vi "Drive Global.vi"() -> ()   [LabVIEW 2014]
panel:
  in  "drive":cluster{"Eje 0":dbl, "Eje 1":dbl, "Eje 2":dbl}
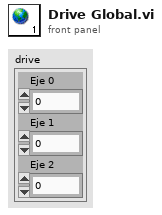
[diagram p1: front panel]
diagram:
